vi "Configure-framegrabber.vi"(8 "error in":errorcluster, 11 "Data ref. in":refnum<data-value>) -> (0 "error IO":errorcluster, 3 "Data ref.":refnum<data-value>, 4 "Initialized?":bool, 5 "Succes?":bool)   [LabVIEW 2013, in "CameraVision.lvlib" / "CV-Main.lvclass"]
doc: "This function initializes the framegrabber hardware (the hardware between the camera and the pc).\nThe necessary memory resources are calculated and allocated.\nThe configuration settings for the framegrabber are loaded from the user selected configuration file and updated with the parameter values from the GUI controls.\n\nSeparate error messages are displayed when either the user selected framegrabber configuration file is corrupted or when the communication to the framegrabber fails."
uses:
  CV-Main.lvclass
  CV-Main.lvclass/CV-Main.ctl
  UI/Module-states.ctl
  UI/Popup-messages.ctl
  Read Config params.vi
  Read Storage params.vi
  Read Acquis params.vi
  Configuration/CV-Configuration.lvclass
  Storage/CV-Storage.lvclass
  Acquisition/CV-Acquisition.lvclass
  UI/CV-UI.lvclass
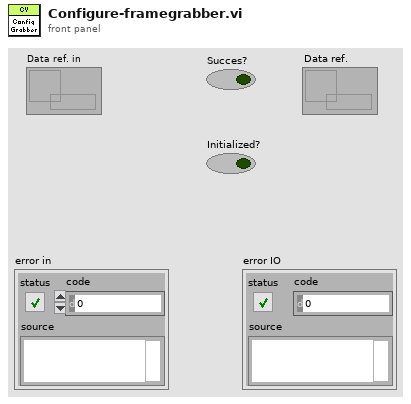
[diagram p1: front panel]
types:
  T1 = typedef "CameraVision.lvlib/CV-UI.lvclass/Module-states.ctl" = enum16{"Inactive", "Active", "Data-loss", "Error", "Simulation", "Synchronizing", "Initialized", "Released"}
  T2 = typedef "CameraVision.lvlib/CV-UI.lvclass/Popup-messages.ctl" = enum16{"Error-Black image", "Error-Camera config file", "Error-Camera connect", "Error-Grabber init", "Error-Camera setting", "Error-Image offset", "Error-Image import", "Error-Settings file not exist", "Error-Timing source", "Conflict-Filters", "Conflict-Map", "Conflict-Framerate", "Conflict-Charact", "Conflict-Temperature field", "Conflict-Temperature value", "Conflict-Storage-Binary image", "Conflict-Storage-Corrected image", "Conflict-Storage-Map", "Conflict-Storage-Charact", "Conflict-Storage-Temperature field", "Conflict-Storage-Temperature value", "Warning-File exist", "Warning-Parameter reset", "Warning-User cancel", "Info-Images imported"}
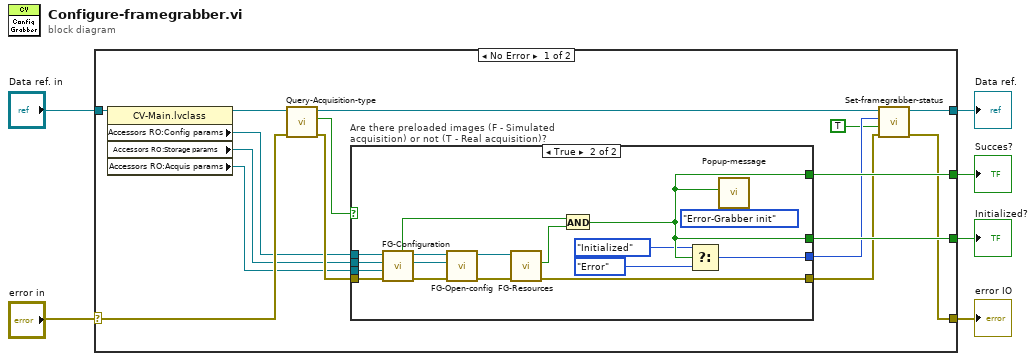
[diagram p0: block diagram]
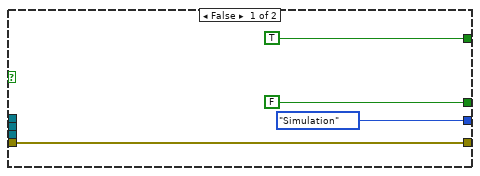
[diagram p2: hidden frame]
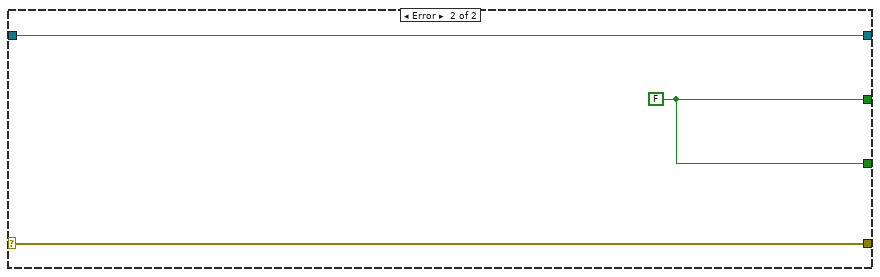
[diagram p3: hidden frame]
diagram:
  n1 = case shown="No Error" "error in" {
    selector: "error in" -> [w18 w46]
    tunnel: [w21 w45] -> w6
    tunnel: [w12 w46] -> w5
    tunnel: [w22 w45] -> w3
    tunnel: "Data ref. in" -> [w20 w44]
    tunnel: [w13 w44] -> w1
    frame No Error {
      n2 = property class="CV-Main.lvclass"(reference=w20) -> (reference out=w19:refnum<data-value>, "Accessors RO:Config params"=w14:refnum<data-value>, "Accessors RO:Storage params"=w8:refnum<data-value>, "Accessors RO:Acquis params"=w7:refnum<data-value>)  [unwired: 1 in, 1 out]
      n3 = call "Query-Acquisition-type.vi"("error in"=w18, "Data ref. in"=w19) -> ("error IO"=w17:errorcluster, "Hardware acquisiton?"=w16:bool, "Data ref."=w15:refnum<data-value>)  [unwired: 7 in]
      n4 = case "Are there preloaded images (F - Simulated acquisition) or not (T - Real acquisition)?" shown="True" w16 {
        tunnel: [FALSE w42] -> w22
        tunnel: [w23 w33] -> w11
        tunnel: [TRUE ("Succes?") w42] -> w21
        tunnel: w14 -> [_ w35]
        tunnel: w17 -> [w23 w34]
        tunnel: [Module-states."Simulation" ("Grabber status") w32] -> w10
        tunnel: w8 -> [_ w30]
        tunnel: w7 -> [_ w31]
        frame False {
        }
        frame True {
          n5 = call "FG-Configuration.vi"("error in"=w34, "Acquis. params. ref."=w31, "Storage params in"=w30, "Config. params. ref."=w35) -> ("error IO"=w36:errorcluster, "Storage params"=w28:refnum<data-value>, "Config. params. ref."=w39:refnum<data-value>, "Succes?"=w29:bool)  [unwired: 4 in]
          n6 = call "FG-Open-config.vi"("error in"=w36, "Storage params"=w28, "Config. params. ref. in"=w39) -> ("error IO"=w37:errorcluster, "Config. params. ref."=w38:refnum<data-value>)  [unwired: 7 in]
          n7 = call "FG-Resources.vi"("error in"=w37, "Config. params. ref. in"=w38) -> ("error IO"=w33:errorcluster, "Succes?"=w43:bool)  [unwired: 7 in, 1 out]
          n8 = And(x=w29, y=w43) -> (x .and. y?=w42:bool)
          n9 = Select(t=Module-states."Initialized", s=w42, f=Module-states."Error" ("Grabber status")) -> (s? t:f=w32:T1)
          n10 = call "Popup-message.vi"("Message"=Popup-messages."Error-Grabber init", "Ignore?"=w42) -> ()  [unwired: 9 in, 1 out]
        }
      }
      n11 = call "Set-framegrabber-status.vi"("error in"=w11, "Reset errors?"=TRUE, "Grabber status in"=w10, "Data ref. in"=w15) -> ("error IO"=w12:errorcluster, "Data ref."=w13:refnum<data-value>)  [unwired: 5 in, 1 out]
    }
    frame Error {
      w45 = FALSE
    }
  }
  "Succes?" <- w6
  "error IO" <- w5
  "Initialized?" <- w3
  "Data ref." <- w1
